vi "initializeArrayElement.vi"(8 "error in (no error)":errorcluster, 9 "arraySize":u16, 10 "arrayRef":refnum<vi>, 11 "String in":refnum<class "String.lvclass">) -> (0 "error out":errorcluster, 3 "String out":refnum<class "String.lvclass">)   [LabVIEW 2016, in "String.lvclass"]
uses:
  String.lvclass
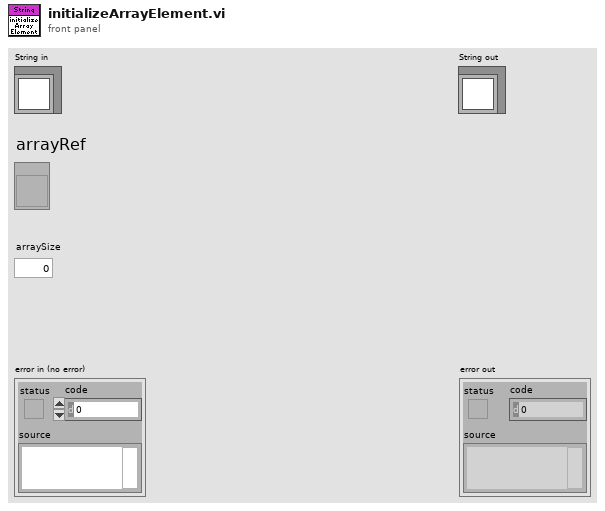
[diagram p1: front panel]
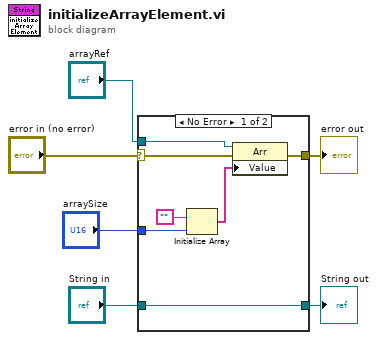
[diagram p0: block diagram]
diagram:
  n1 = case shown="No Error" "error in (no error)" {
    selector: "error in (no error)" -> [w12 w15]
    tunnel: [w11 w15] -> w3
    tunnel: "arraySize" -> [w10 _]
    tunnel: [w9 w14] -> w5
    tunnel: "String in" -> [w9 w14]
    tunnel: "arrayRef" -> [w8 _]
    frame No Error {
      n2 = Initialize Array("", w10) -> (w13:string[])
      n3 = property class="Arr"(reference=w8, error in=w12, "Value"=w13) -> (error out=w11:errorcluster)  [unwired: 1 out]
    }
    frame Error {
    }
  }
  "error out" <- w3
  "String out" <- w5
